vi "Imaq_to_pythonArray.vi"(8 "error in (no error)":errorcluster, 10 "input(RGB_U32)":T1, 11 "output ref name":string="image_output") -> (0 "error out":errorcluster, 1 "Image Out":T1, 2 "image_in":T1, 3 "python_image":u8[][][](array[numeric]), 4 "elapsed_time":u32)   [LabVIEW 2021]
uses:
  <vilib>/vision/Image Controls.llb/IMAQ Image.ctl
  <vilib>/vision/NI_Vision_Development_Module.lvlib
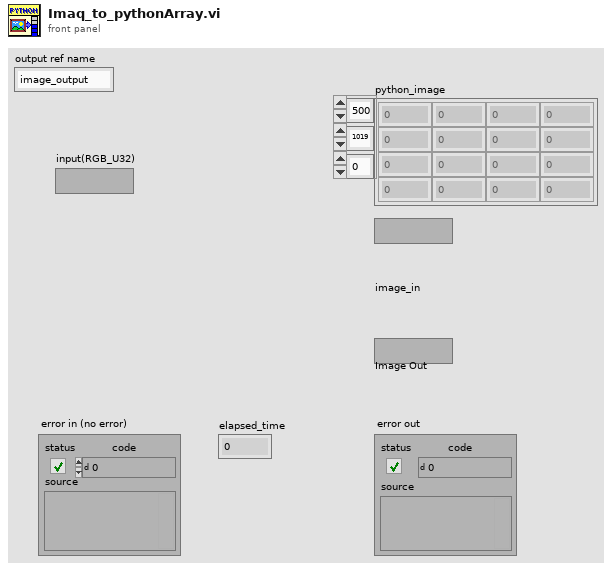
[diagram p1: front panel]
types:
  T1 = typedef "IMAQ Image.ctl" = refnum<image>
  T2 = typedef "Image Type" = u32
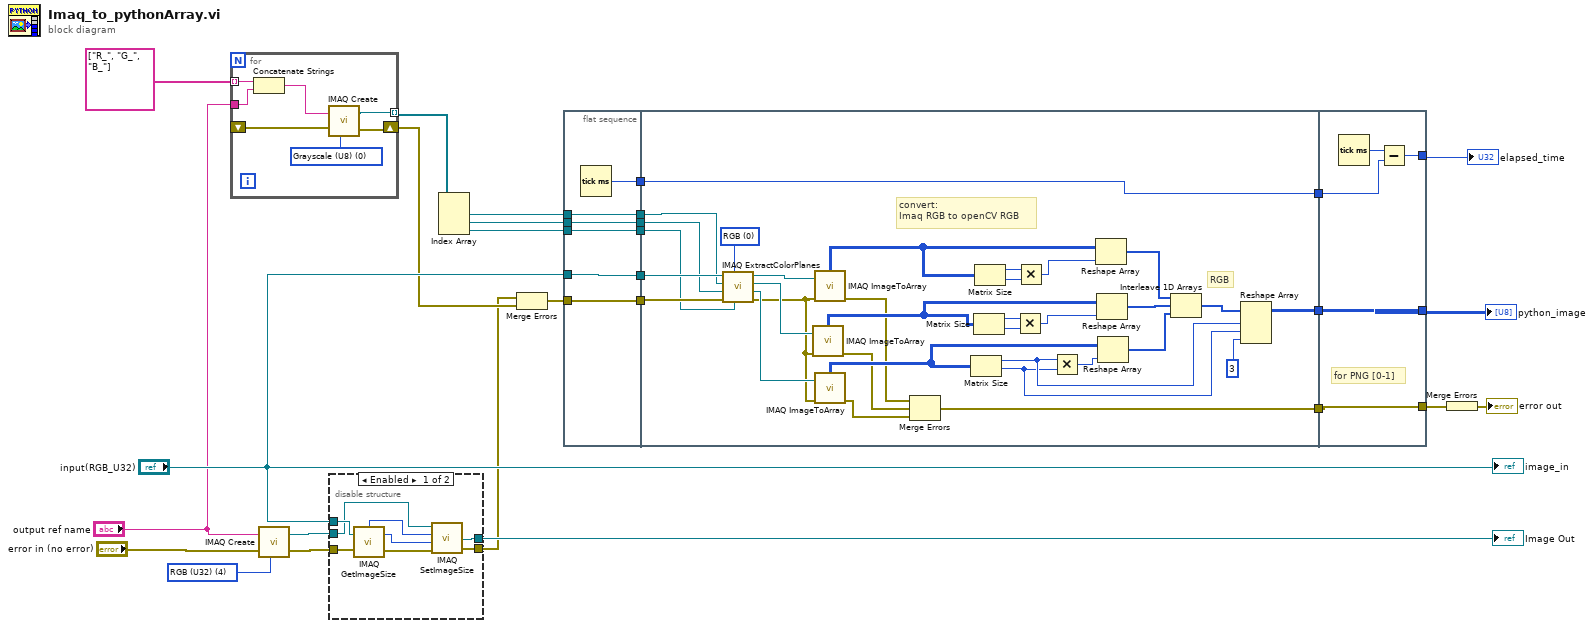
[diagram p0: block diagram]
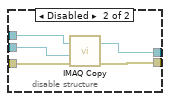
[diagram p2: hidden frame]
diagram:
  w13 = T2 4 items=["Grayscale (U8)", "Grayscale (I16)", "Grayscale (SGL)", "Complex (CSG)", "RGB (U32)", "HSL (U32)", "RGB (U64)", "Grayscale (U16)"] ("Image Type")
  n1 = for {
    tunnel: string[] ["R_", "G_", "B_"] ("Image Name 2") -> [w34] mode=indexing
    shift-right: [w32] -> w3
    shift-left: _ -> [w33]
    tunnel: [w31] -> w10 mode=indexing
    tunnel: "output ref name" -> [w29]
    w35 = T2 0 items=["Grayscale (U8)", "Grayscale (I16)", "Grayscale (SGL)", "Complex (CSG)", "RGB (U32)", "HSL (U32)", "RGB (U64)", "Grayscale (U16)"] ("Image Type")
    n2 = Concatenate Strings(w34, w29) -> (w30:string)
    n3 = call "IMAQ Create"("Image Name"=w30, "Image Type"=w35, "error in (no error)"=w33) -> ("New Image"=w31:T1, "error out"=w32:errorcluster)  [unwired: 2 in]
  }
  n4 = call "IMAQ Create"("Image Name"="output ref name", "Image Type"=w13, "error in (no error)"="error in (no error)") -> ("New Image"=w12:T1, "error out"=w6:errorcluster)  [unwired: 2 in]
  n5 = disable-structure shown="Enabled" {
    disable-tunnel: [w41 w44] -> w20
    disable-tunnel: "input(RGB_U32)" -> [w39 w46]
    disable-tunnel: w12 -> [w38 w45]
    disable-tunnel: w6 -> [w37 w48]
    disable-tunnel: [w36 w47] -> w2
    frame Enabled {
      n6 = call "IMAQ GetImageSize"("Image"=w39, "error in (no error)"=w37) -> ("Y Resolution"=w42:i32, "X Resolution"=w43:i32, "error out"=w40:errorcluster)  [unwired: 2 in]
      n7 = call "IMAQ SetImageSize"("error in (no error)"=w40, "Y Resolution"=w42, "X Resolution"=w43, "Image"=w38) -> ("error out"=w36:errorcluster, "Image Out"=w41:T1)  [unwired: 1 in]
    }
    frame Disabled {
      n8 = call "IMAQ Copy"("error in (no error)"=w48, "Image Dst"=w45, "Image Src"=w46) -> ("error out"=w47:errorcluster, "Image Dst Out"=w44:T1)  [unwired: 3 in]
    }
  }
  "Image Out" <- w20
  n9 = Index Array(array=w10) -> (element #1=w7:T1, element #2=w8:T1, element #3=w9:T1)  [unwired: 3 in]
  n10 = Merge Errors(w2, w3) -> (w4:errorcluster)
  n11 = flat-sequence {
    tunnel: "input(RGB_U32)" -> [w53]
    tunnel: w4 -> [w54]
    tunnel: [w54] -> w28
    tunnel: [w53] -> w27
    tunnel: [w52] -> w26
    tunnel: [w51] -> w25
    tunnel: w7 -> [w51]
    tunnel: [w50] -> w24
    tunnel: w8 -> [w50]
    tunnel: [w49] -> w23
    tunnel: w9 -> [w49]
    tunnel: w28 -> [w82]
    tunnel: w27 -> [w81]
    tunnel: [w84] -> w22
    tunnel: [w83] -> w21
    tunnel: w26 -> [w83]
    tunnel: w25 -> [w80]
    tunnel: w24 -> [w79]
    tunnel: w23 -> [w78]
    tunnel: [w75] -> w16
    tunnel: [w89] -> w19
    tunnel: w22 -> [w89]
    tunnel: w21 -> [w91]
    tunnel: [w90] -> w18
    tunnel: [w88] -> w17
    tunnel: w16 -> [w88]
    frame #0 {
      n12 = Tick Count (ms)() -> (millisecond timer value=w52:u32)
    }
    frame #1 {
      w71 = u16 0 items=["RGB", "HSL", "HSV", "HSI"] ("Color Mode")
      # "convert:\nImaq RGB to openCV RGB"
      # "RGB"
      n13 = call "IMAQ ExtractColorPlanes"("Blue or Luma or Val or Inten Plane"=w78, "Color Mode"=w71, "error in (no error)"=w82, "Green or Sat Plane"=w79, "Red or Hue Plane"=w80, "Image Src"=w81) -> ("error out"=w60:errorcluster, "Blue or Luma or Val or Inten Plane out"=w72:T1, "Green or Sat Plane out"=w73:T1, "Red or Hue Plane out"=w74:T1)  [unwired: 2 in]
      n14 = call "IMAQ ImageToArray"("error in (no error)"=w60, "Image"=w73) -> ("error out"=w57:errorcluster, "Image Pixels (U8)"=w61:u8[][])  [unwired: 2 in, 3 out]
      n15 = call "IMAQ ImageToArray"("error in (no error)"=w60, "Image"=w74) -> ("error out"=w58:errorcluster, "Image Pixels (U8)"=w70:u8[][])  [unwired: 2 in, 3 out]
      n16 = call "IMAQ ImageToArray"("error in (no error)"=w60, "Image"=w72) -> ("error out"=w59:errorcluster, "Image Pixels (U8)"=w62:u8[][])  [unwired: 2 in, 3 out]
      n17 = Merge Errors(w58, w57, w59) -> (w75:errorcluster)
      n18 = Matrix Size(0:w62) -> (1:w77:i32, 2:w76:i32)
      n19 = Matrix Size(0:w61) -> (1:w65:i32, 2:w66:i32)
      n20 = Matrix Size(0:w70) -> (1:w69:i32, 2:w68:i32)
      n21 = Multiply(x=w65, y=w66) -> (x*y=w64:i32)
      n22 = Multiply(x=w69, y=w68) -> (x*y=w67:i32)
      n23 = Multiply(x=w77, y=w76) -> (x*y=w63:i32)
      n24 = Reshape Array(w70, w67) -> (w87:u8[])
      n25 = Reshape Array(w61, w64) -> (w86:u8[])
      n26 = Reshape Array(w62, w63) -> (w85:u8[])
      n27 = Interleave 1D Arrays(w87, w86, w85) -> (w56:u8[])
      n28 = Reshape Array(w56, w77, w76, 3 ("dimension size")) -> (w84:u8[][][])
    }
    frame #2 {
      # "for PNG [0-1]"
      n29 = Tick Count (ms)() -> (millisecond timer value=w92:u32)
      n30 = Subtract(x=w92, y=w91) -> (x-y=w90:u32)
    }
  }
  n31 = Merge Errors(w17) -> (→"error out":errorcluster)
  "image_in" <- "input(RGB_U32)"
  "python_image" <- w19
  "elapsed_time" <- w18
